vi "PID.vi"(0 "当前值":dbl, 1 "kp":dbl, 2 "ki":dbl, 3 "kd":dbl, 4 "目标值":dbl) -> (5 "输出值":dbl)   [LabVIEW 2018]
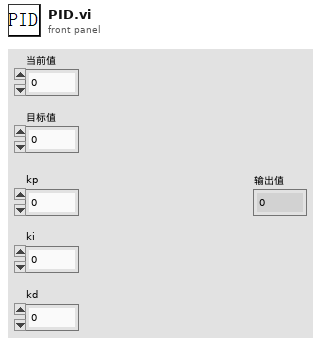
[diagram p1: front panel]
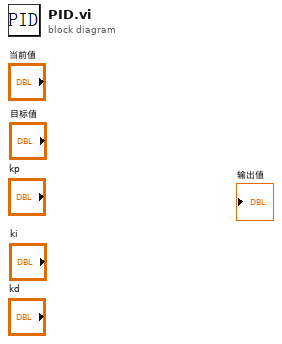
[diagram p0: block diagram]
diagram:
